vi "DAQ_Thermometer.vi"() -> ()   [LabVIEW 2020]
panel:
  in  "file path (use dialog)":path
  in  "Number of sample":dbl
  out "Waveform Chart":dbl[](graph)
  out "Array 2":dbl[](array[numeric])
  out "Array":dbl[](array[knob]) scale=0.0..100.0
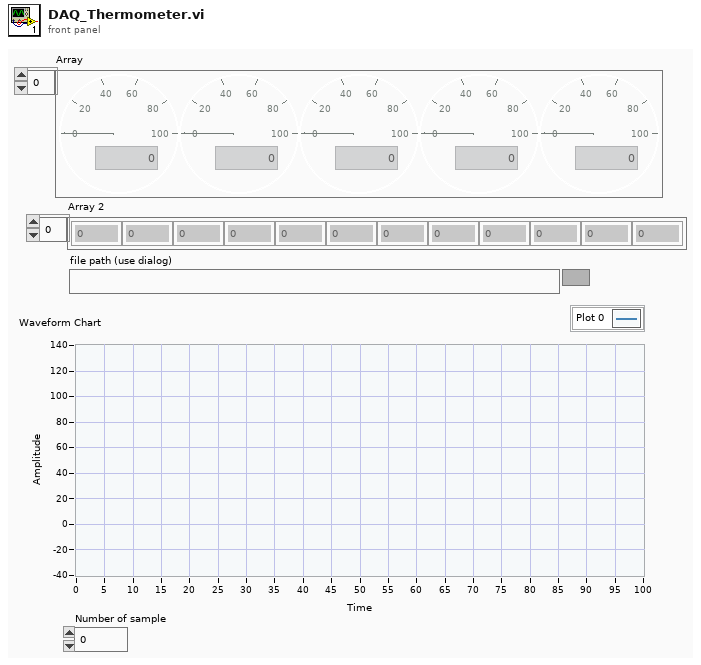
[diagram p1: front panel]
types:
  T1 = enum16{"open", "replace", "create", "open or create", "replace or create", "replace or create with confirmation"}
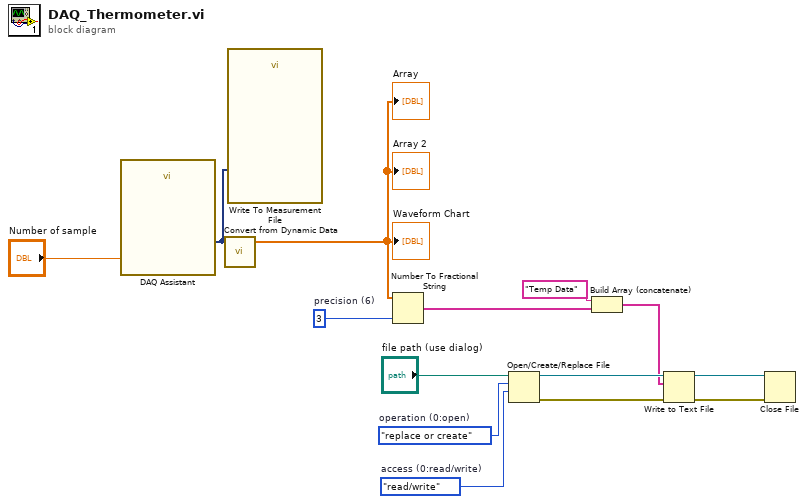
[diagram p0: block diagram]
diagram:
  w4 = i16 3  # precision (6)
  w6 = T1."replace or create"  # operation (0:open)
  w7 = enum16{"read/write", "read-only", "write-only"}."read/write"  # access (0:read/write)
  n1 = call "DAQ Assistant"("number of samples"="Number of sample") -> ("data"=w13:dynamicdata)  [unwired: 16 in, 2 out]
  n2 = call "Convert from Dynamic Data"("Dynamic Data Type"=w13) -> ("Array"=w5:dbl[])  [unwired: 3 in]
  "Array" <- w5
  "Array 2" <- w5
  "Waveform Chart" <- w5
  n3 = call "Write To Measurement File"("Signals"=w13) -> ()  [unwired: 16 in, 3 out]
  n4 = Number To Fractional String(number=w5, precision (6)=w4) -> (F-format string=w3:string[])  [unwired: 2 in]
  n5 = Open/Create/Replace File(file path (use dialog)="file path (use dialog)", operation (0:open)=w6, access (0:read/write)=w7) -> (refnum out=w12:refnum<file>, error out=w10:errorcluster)  [unwired: 3 in, 1 out]
  n6 = Build Array (concatenate) "Build Array"("Temp Data", w3) -> (w1:string[])
  n7 = Write to Text File(file (use dialog)=w12, text=w1, error in=w10) -> (refnum out=w11:refnum<file>, error out=w9:errorcluster)  [unwired: 1 in, 1 out]
  n8 = Close File(refnum=w11, error in=w9) -> ()  [unwired: 2 out]
